vi "Init.vi"(6 "Harmonic":i8, 8 "error in (no error)":errorcluster, 9 "SA Pin":string, 10 "Measurement Name":string, 11 "Standard":string) -> (0 "error out":errorcluster, 3 "Harmonics_CHP out":refnum<class "Harmonics_CHP.lvclass">)   [LabVIEW 2016, in "SeqAuto Evaluations.lvlib" / "Harmonics_CHP.lvclass"]
uses:
  Harmonics_CHP.lvclass
  C:/projects/STS/Common/Sequence Automation/Plugins/SeqAuto IEvaluation.lvlibp/SeqAuto IEvaluation.lvclass
  Harmonics_CHP.lvclass/Harmonics_CHP.ctl
  Write Harmonic.vi
  Write SA Pin.vi
  Plugins/SeqAuto IEvaluation.lvlibp/Write Measurement Name.vi
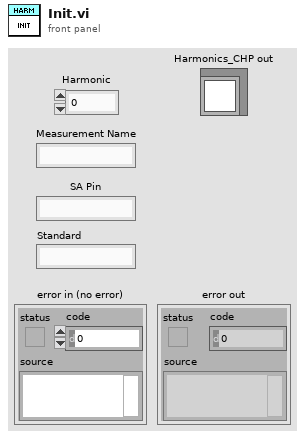
[diagram p1: front panel]
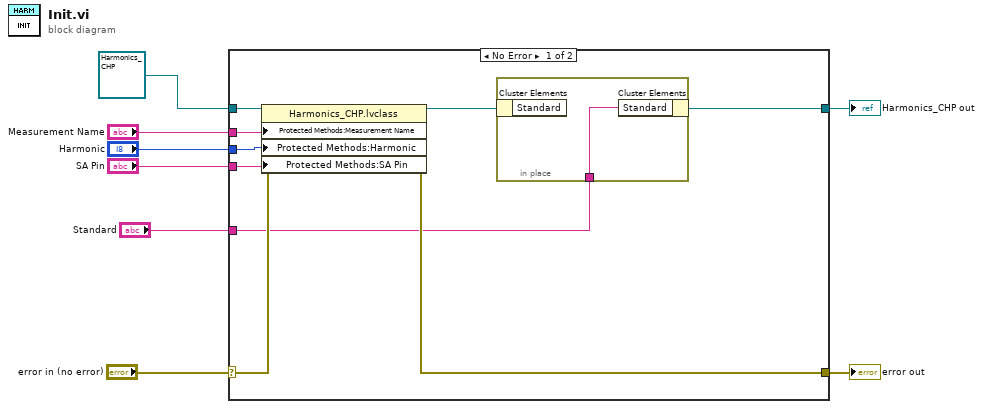
[diagram p0: block diagram]
diagram:
  n1 = case shown="No Error" "error in (no error)" {
    selector: "error in (no error)" -> [w17 w20]
    tunnel: [w16 w20] -> w7
    tunnel: [w10 w19] -> w5
    tunnel: refnum<class "Harmonics_CHP.lvclass"> refnum ("Harmonics_CHP in") -> [w15 w19]
    tunnel: "Measurement Name" -> [w14 _]
    tunnel: "Harmonic" -> [w13 _]
    tunnel: "SA Pin" -> [w12 _]
    tunnel: "Standard" -> [w9 _]
    frame No Error {
      n2 = property class="Harmonics_CHP.lvclass"(reference=w15, error in=w17, "Protected Methods:Measurement Name"=w14, "Protected Methods:Harmonic"=w13, "Protected Methods:SA Pin"=w12) -> (reference out=w11:refnum<class "Harmonics_CHP.lvclass">, error out=w16:errorcluster)
      n3 = in-place {
        in-place-border: w9 -> [w18]
        n4 = in-place-cluster #1(w11) -> ()  [unwired: 1 out]
        n5 = in-place-cluster #1("Standard"=w18) -> (w10:refnum<class "Harmonics_CHP.lvclass">)
      }
    }
    frame Error {
    }
  }
  "error out" <- w7
  "Harmonics_CHP out" <- w5
